vi "ExpStateLoadBridge.vi"(3 "Error In":errorcluster, 5 "Experiment State IN":T1={"error"={"status"=FALSE, "code"=0, "source"=""}, "Digitizer DAQmx Tasks"={"TaskArray"=[]}, "Digitizer Settings"={"Channel Settings"=[], "Card Settings"=[]}, "Synchronization Settings"={"Synchronizer"="PXI1Slot2", "source terminal"="GlobalSoftwareTrigger"}, "Digitizer Data"=[], "Next Shot#"="0", "System Message"="", "User Shot Notes"="", "Timing Settings"={"Timing Card Settings"=[], "Timing Channel Settings"=[[{"Delay (s)"=2.559999942779541, "Pulse width (s)"=0.009999999776482582, "Active"=TRUE, "Channel Name"="Fiber 8", "counter"="PXI1Slot8/ctr7", "FrontPanelTime"=2.559999942779541}]]}, "Timing Tasks"={"TaskArray"=[]}, "Tree"="0", "Time Card/Channels"=[2, 8], "DAQ Card/Channels"=[3, 8], "Program Version"=""} {"Timing Settings"."Timing Channel Settings"."FrontPanelTime" format="%.3p"; "Timing Settings"."Timing Channel Settings"."Pulse width (s)" format="%.3p"; "Timing Settings"."Timing Channel Settings"."Delay (s)" format="%.3p"; "Digitizer Settings"."Card Settings"."Global Edge Type" items=["Rising"=10280, "Falling"=10171]; "Digitizer Settings"."Card Settings"."Sample Rate" format="%#_3p"}) -> (0 "Initialized DAQ Array":T11(array[cluster]) {"Card Settings"."Start Time" format="%#_3p"; "Card Settings"."End Time" format="%#_3p"; "Card Settings"."Rate" format="%#_3p"}, 1 "Initialized Timing Array":T12[](array[typedef]) {"Timing Sequence"."Dt" format="%_3p"; "Timing Sequence"."Time" format="%_3p"}, 2 "Experiment State OUT":T1={"error"={"status"=FALSE, "code"=0, "source"=""}, "Digitizer DAQmx Tasks"={"TaskArray"=[]}, "Digitizer Settings"={"Channel Settings"=[], "Card Settings"=[]}, "Synchronization Settings"={"Synchronizer"="PXI1Slot2", "source terminal"="GlobalSoftwareTrigger"}, "Digitizer Data"=[], "Next Shot#"="0", "System Message"="", "User Shot Notes"="", "Timing Settings"={"Timing Card Settings"=[], "Timing Channel Settings"=[[{"Delay (s)"=2.559999942779541, "Pulse width (s)"=0.009999999776482582, "Active"=TRUE, "Channel Name"="Fiber 8", "counter"="PXI1Slot8/ctr7", "FrontPanelTime"=2.559999942779541}]]}, "Timing Tasks"={"TaskArray"=[]}, "Tree"="0", "Time Card/Channels"=[2, 8], "DAQ Card/Channels"=[3, 8], "Program Version"=""} {"Timing Settings"."Timing Channel Settings"."FrontPanelTime" format="%.3p"; "Timing Settings"."Timing Channel Settings"."Pulse width (s)" format="%.3p"; "Timing Settings"."Timing Channel Settings"."Delay (s)" format="%.3p"; "Digitizer Settings"."Card Settings"."Global Edge Type" items=["Rising"=10280, "Falling"=10171]; "Digitizer Settings"."Card Settings"."Sample Rate" format="%#_3p"})   [LabVIEW 2013]
uses:
  Controls/TimingControl.ctl
  Controls/TimingControlChannel.ctl
  Controls/DAQ Card Channel Array.ctl
  Controls/DAQ Channel Settings.ctl
  Controls/DAQ Card Settings.ctl
  Controls/ExperimentStateCluster.ctl
  Controls/DigitizerSettingsChannelSettings.ctl
  Controls/DigitizerSettingsCardSettingsArray.ctl
  Controls/DigitizerSettingsCardSettings.ctl
  Controls/TimingSettings.ctl
  Controls/TimingCardSettings.ctl
  Controls/TimingChannelSettings.ctl
  Controls/DAQ Card-Channel Settings.ctl
panel:
  # "Sampling Rate [1/s]"
  # "Start Time [s]"
  # "End Time [s]"
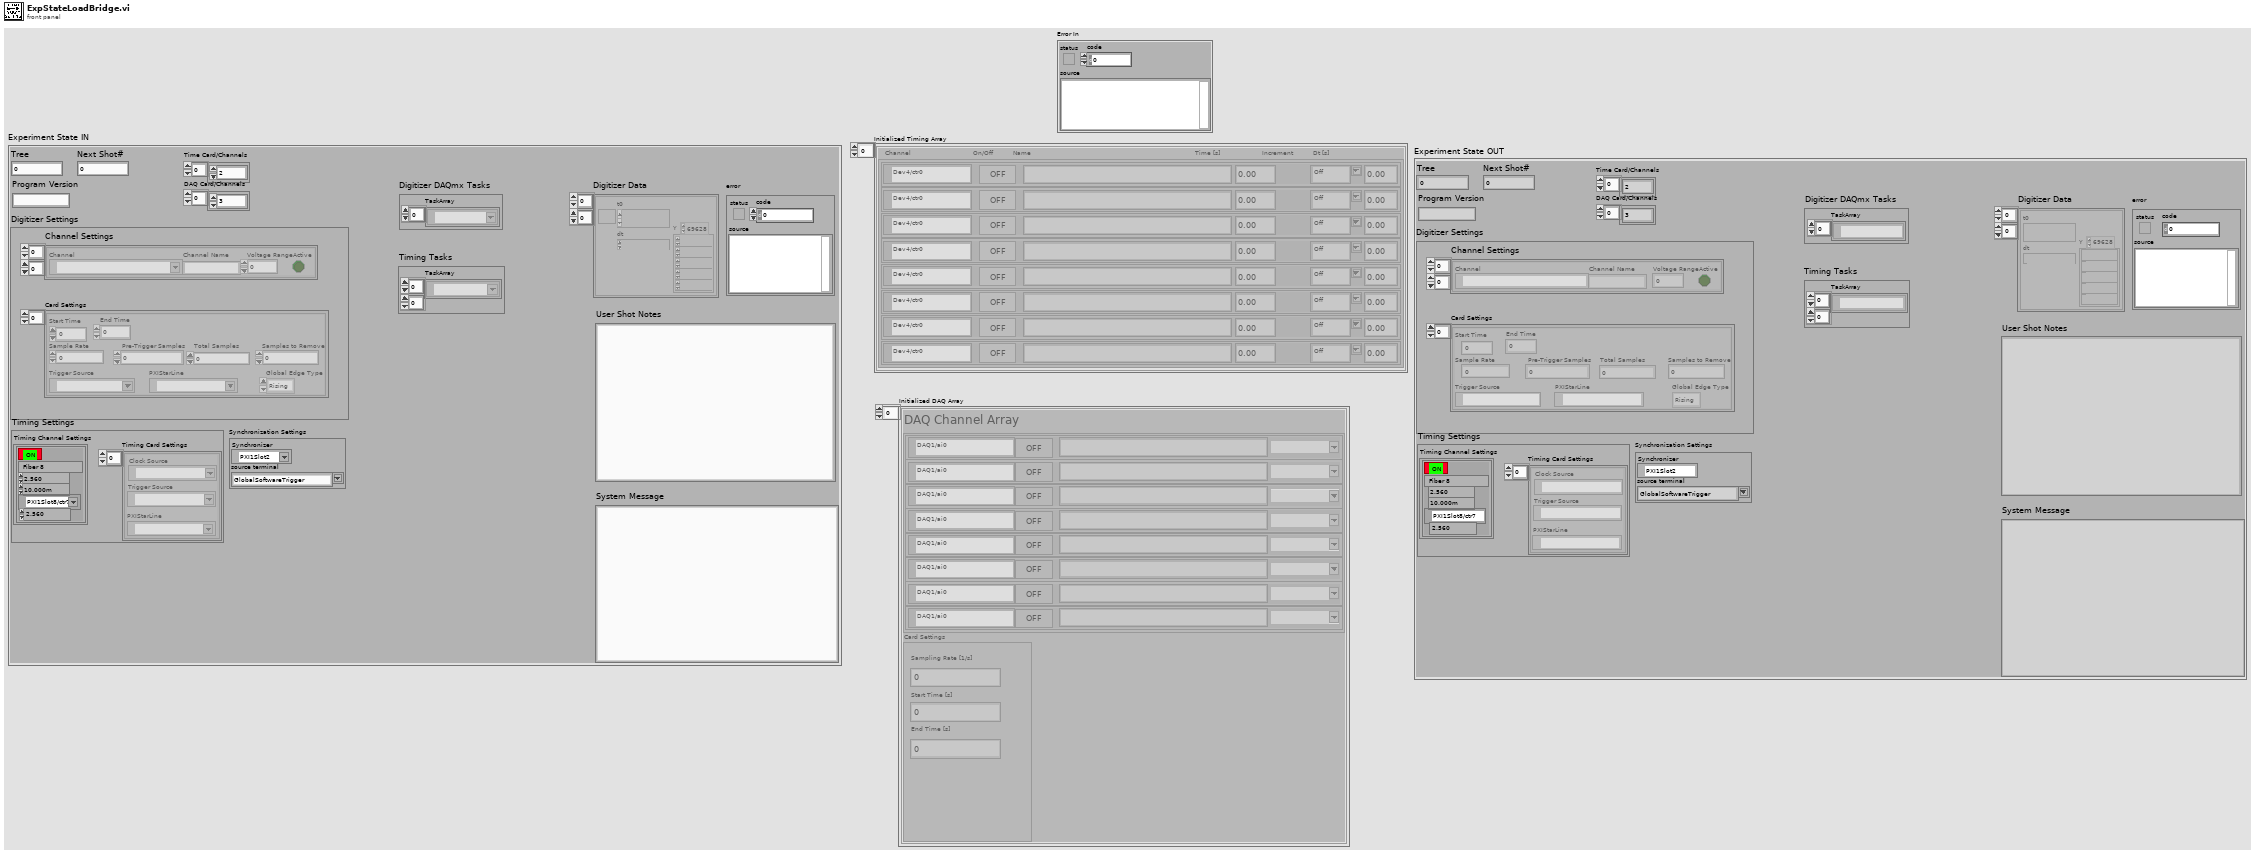
[diagram p1: front panel]
types:
  T1 = typedef "ExperimentStateCluster.ctl" = cluster{"error":errorcluster, "Digitizer DAQmx Tasks":cluster{"TaskArray":refnum<k21>[]}, "Digitizer Settings":cluster{"Channel Settings":T2[][], "Card Settings":T3}, "Synchronization Settings":cluster{"Synchronizer":refnum<k15>, "source terminal":string}, "Digitizer Data":waveform(dbl)[][], "Next Shot#":string, "System Message":string, "User Shot Notes":string, "Timing Settings":T5, "Timing Tasks":cluster{"TaskArray":refnum<k21>[][]}, "Tree":string, "Time Card/Channels":i32[], "DAQ Card/Channels":i32[], "Program Version":string}
  T2 = typedef "DigitizerSettingsChannelSettings.ctl" = cluster{"Channel":tag, "Channel Name":string, "Voltage Range":dbl, "Active":bool}
  T3 = typedef "DigitizerSettingsCardSettingsArray.ctl" = T4[]
  T4 = typedef "DigitizerSettingsCardSettings.ctl" = cluster{"Start Time":dbl, "End Time":dbl, "Sample Rate":dbl, " Pre-Trigger Samples":u32, "Total Samples":i32, "Samples to Remove":u32, "Trigger Source":tag, "Global Edge Type":i32, "PXIStarLine":tag}
  T5 = typedef "TimingSettings.ctl" = cluster{"Timing Card Settings":T6[], "Timing Channel Settings":T7[][]}
  T6 = typedef "TimingCardSettings.ctl" = cluster{"Trigger Source":tag, "Clock Source":tag, "PXIStarLine":tag}
  T7 = typedef "TimingChannelSettings.ctl" = cluster{"Delay (s)":dbl, "Pulse width (s)":dbl, "Active":bool, "Channel Name":string, "counter":tag, "FrontPanelTime":dbl}
  T8 = typedef "DAQ Card Channel Array.ctl" = T9[]
  T9 = typedef "DAQ Channel Settings.ctl" = cluster{"Active":bool, "Channel Name":string, "Channel":tag, "Voltage Range":string}
  T10 = typedef "DAQ Card Settings.ctl" = cluster{"Rate":dbl, "End Time":dbl, "Start Time":dbl}
  T11 = cluster{"DAQ Channel Array":T8, "Card Settings":T10}[]
  T12 = typedef "TimingControl.ctl" = cluster{"Timing Sequence":T13[]}
  T13 = typedef "TimingControlChannel.ctl" = cluster{"Active":bool, "counter":tag, "Channel Name":string, "Time":dbl, "Increment":string, "Dt":dbl}
  T14 = typedef "DAQ Card-Channel Settings.ctl" = cluster{"DAQ Channel Array":T8, "Card Settings":T10}
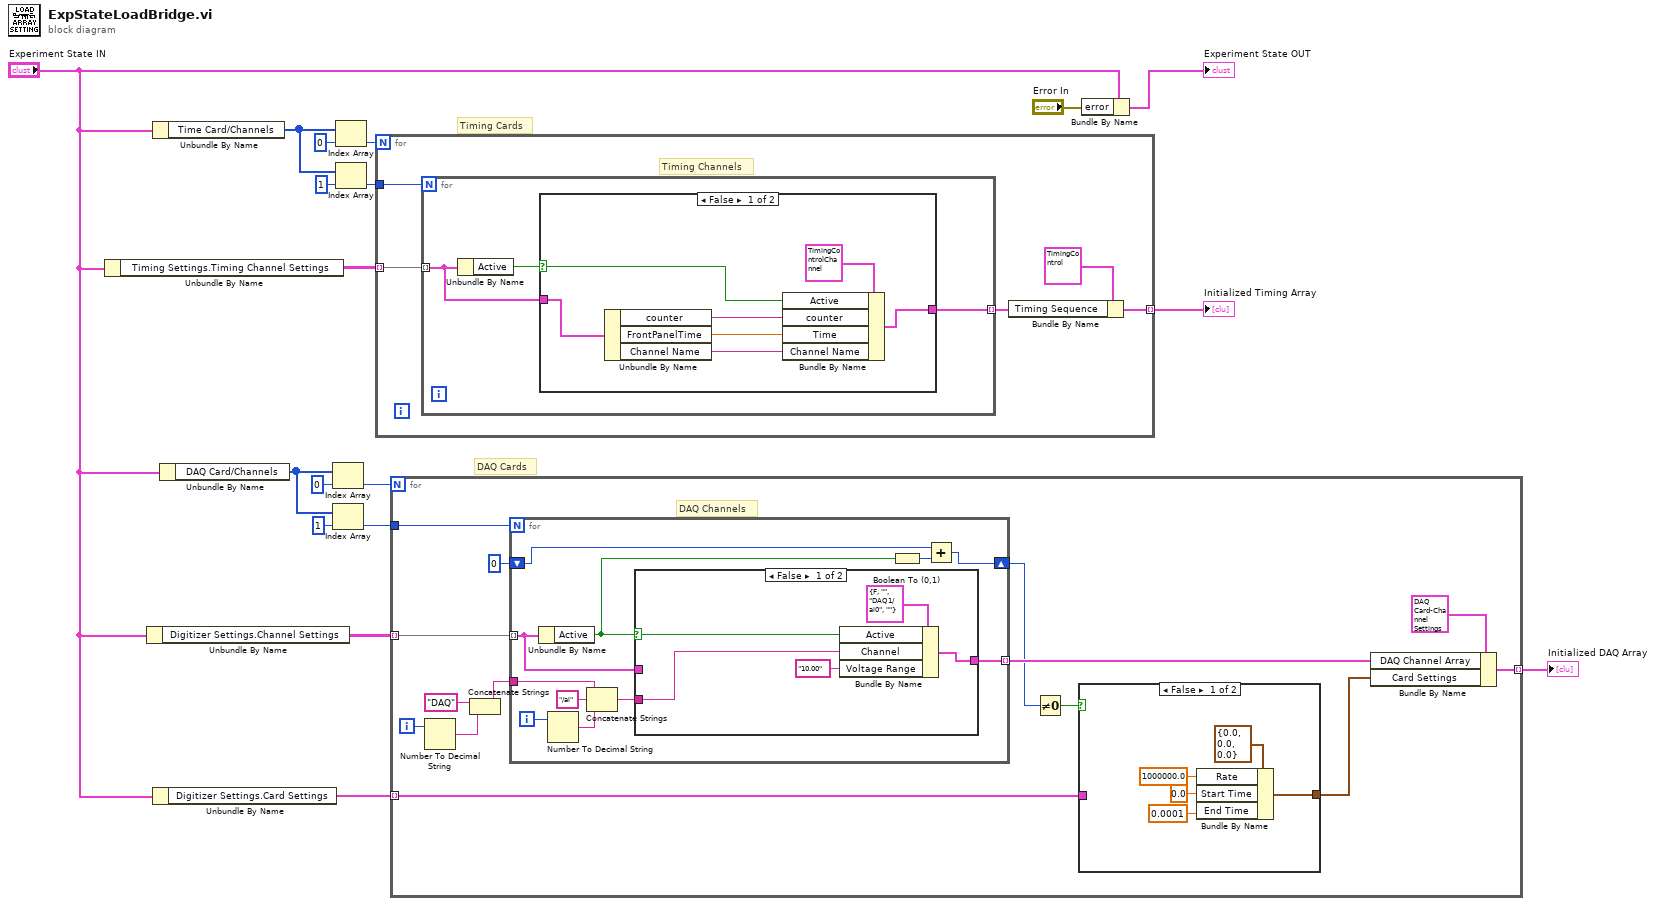
[diagram p0: block diagram]
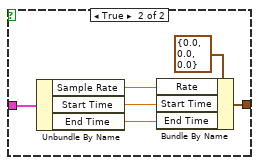
[diagram p2: hidden frame]
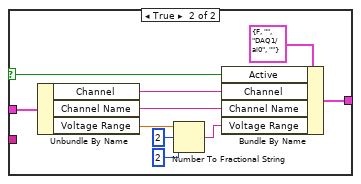
[diagram p3: hidden frame]
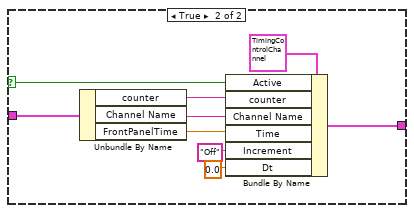
[diagram p4: hidden frame]
diagram:
  # "DAQ Cards"
  # "Timing Cards"
  n1 = Unbundle By Name("Experiment State IN") -> ("Timing Settings.Timing Channel Settings"=w11:T7[][])
  n2 = Unbundle By Name("Experiment State IN") -> ("Digitizer Settings.Channel Settings"=w5:T2[][])
  n3 = Unbundle By Name("Experiment State IN") -> ("Time Card/Channels"=w13:i32[])
  n4 = Unbundle By Name("Experiment State IN") -> ("Digitizer Settings.Card Settings"=w4:T3)
  n5 = Unbundle By Name("Experiment State IN") -> ("DAQ Card/Channels"=w8:i32[])
  n6 = Index Array(array=w8, index=0) -> (element=w7:i32)
  n7 = Index Array(array=w8, index=1) -> (element=w6:i32)
  n8 = Index Array(array=w13, index=0) -> (element=w16:i32)
  n9 = Index Array(array=w13, index=1) -> (element=w12:i32)
  n10 = for {
    N: w16 -> [_]
    tunnel: [w23] -> w18 mode=indexing
    tunnel: w12 -> [w20]
    tunnel: w11 -> [w19] mode=indexing
    # "Timing Channels"
    n11 = for {
      N: w20 -> [_]
      tunnel: [w25] -> w21 mode=indexing
      tunnel: w19 -> [w24] mode=indexing
      n12 = Unbundle By Name(w24) -> ("Active"=w26:bool)
      n13 = case shown="False" w26 {
        selector: w26 -> [w32 w38]
        tunnel: [w31 w39] -> w25
        tunnel: w24 -> [w30 w37]
        frame False {
          n14 = Unbundle By Name(w30) -> ("counter"=w29:tag, "FrontPanelTime"=w28:dbl, "Channel Name"=w27:string)
          n15 = Bundle By Name(cluster=T13 {"Active"=FALSE, "counter"="PXI1Slot9/ctr7", "Channel Name"="", "Time"=0.0, "Increment"="Off", "Dt"=0.0} ("Counters"), "Active"=w32, "counter"=w29, "Time"=w28, "Channel Name"=w27) -> (w31:T13)
        }
        frame True {
          n16 = Unbundle By Name(w37) -> ("counter"=w36:tag, "Channel Name"=w35:string, "FrontPanelTime"=w34:dbl)
          n17 = Bundle By Name(cluster=T13 {"Active"=FALSE, "counter"="PXI1Slot9/ctr7", "Channel Name"="", "Time"=0.0, "Increment"="Off", "Dt"=0.0} ("Counters"), "Active"=w38, "counter"=w36, "Channel Name"=w35, "Time"=w34, "Increment"="Off", "Dt"=0.0) -> (w39:T13)
        }
      }
    }
    n18 = Bundle By Name(cluster=T12 {"Timing Sequence"=[{"Active"=FALSE, "counter"="PXI1Slot9/ctr7", "Channel Name"="", "Time"=0.0, "Increment"="Off", "Dt"=0.0}, {"Active"=FALSE, "counter"="Dev4/ctr0", "Channel Name"="", "Time"=0.0, "Increment"="Off", "Dt"=0.0}, {"Active"=FALSE, "counter"="Dev4/ctr0", "Channel Name"="", "Time"=0.0, "Increment"="Off", "Dt"=0.0}, {"Active"=FALSE, "counter"="Dev4/ctr0", "Channel Name"="", "Time"=0.0, "Increment"="Off", "Dt"=0.0}, {"Active"=FALSE, "counter"="Dev4/ctr0", "Channel Name"="", "Time"=0.0, "Increment"="Off", "Dt"=0.0}, {"Active"=FALSE, "counter"="Dev4/ctr0", "Channel Name"="", "Time"=0.0, "Increment"="Off", "Dt"=0.0}, {"Active"=FALSE, "counter"="Dev4/ctr0", "Channel Name"="", "Time"=0.0, "Increment"="Off", "Dt"=0.0}, {"Active"=FALSE, "counter"="Dev4/ctr0", "Channel Name"="", "Time"=0.0, "Increment"="Off", "Dt"=0.0}]} ("Cluster"), "Timing Sequence"=w21) -> (w23:T12)
  }
  "Initialized Timing Array" <- w18
  n19 = for {
    N: w7 -> [_]
    tunnel: [w56] -> w17 mode=indexing
    tunnel: w6 -> [w53]
    tunnel: w5 -> [w52] mode=indexing
    tunnel: w4 -> [w47] mode=indexing
    i -> [w44]
    # "DAQ Channels"
    n20 = Number To Decimal String(number=w44) -> (decimal integer string=w46:string)  [unwired: 1 in]
    n21 = Concatenate Strings("DAQ", w46) -> (w43:string)
    n22 = for {
      N: w53 -> [_]
      tunnel: [w78] -> w54 mode=indexing
      tunnel: w52 -> [w77] mode=indexing
      shift-right: [w73] -> w49
      shift-left: 0 -> [w74]
      tunnel: w43 -> [w70]
      i -> [w69]
      n23 = Unbundle By Name(w77) -> ("Active"=w75:bool)
      n24 = Number To Decimal String(number=w69) -> (decimal integer string=w72:string)  [unwired: 1 in]
      n25 = Concatenate Strings(w70, "/ai" ("string"), w72) -> (w68:string)
      n26 = case shown="False" w75 {
        selector: w75 -> [w81 w91]
        tunnel: [w82 w93] -> w78
        tunnel: w77 -> [_ w90]
        tunnel: w68 -> [w79 _]
        frame False {
          n27 = Bundle By Name(cluster=T9 {"Active"=FALSE, "Channel Name"="", "Channel"="DAQ1/ai0", "Voltage Range"=""} ("Counters"), "Active"=w81, "Channel"=w79, "Voltage Range"="10.00") -> (w82:T9)
        }
        frame True {
          n28 = Unbundle By Name(w90) -> ("Channel"=w88:tag, "Channel Name"=w89:string, "Voltage Range"=w86:dbl)
          n29 = Number To Fractional String(number=w86, width (-)=i16 2, precision (6)=i16 2) -> (F-format string=w87:string)  [unwired: 1 in]
          n30 = Bundle By Name(cluster=T9 {"Active"=FALSE, "Channel Name"="", "Channel"="DAQ1/ai0", "Voltage Range"=""} ("Counters"), "Active"=w91, "Channel"=w88, "Channel Name"=w89, "Voltage Range"=w87) -> (w93:T9)
        }
      }
      n31 = Boolean To (0,1)(Boolean=w75) -> (0, 1=w76:i16)
      n32 = Add(x=w74, y=w76) -> (x+y=w73:i32)
    }
    n33 = Not Equal To 0?(x=w49) -> (x != 0?=w50:bool)
    n34 = case shown="False" w50 {
      tunnel: [w58 w66] -> w48
      tunnel: w47 -> [_ w65]
      frame False {
        n35 = Bundle By Name(cluster=T10 {"Rate"=0.0, "End Time"=0.0, "Start Time"=0.0} ("Card Settings"), "Rate"=1000000.0, "Start Time"=0.0, "End Time"=0.0001) -> (w58:T10)
      }
      frame True {
        n36 = Unbundle By Name(w65) -> ("Sample Rate"=w62:dbl, "Start Time"=w63:dbl, "End Time"=w64:dbl)
        n37 = Bundle By Name(cluster=T10 {"Rate"=0.0, "End Time"=0.0, "Start Time"=0.0} ("Card Settings"), "Rate"=w62, "Start Time"=w63, "End Time"=w64) -> (w66:T10)
      }
    }
    n38 = Bundle By Name(cluster=T14 {"DAQ Channel Array"=[{"Active"=FALSE, "Channel Name"="", "Channel"="DAQ1/ai0", "Voltage Range"=""}, {"Active"=FALSE, "Channel Name"="", "Channel"="DAQ1/ai0", "Voltage Range"=""}, {"Active"=FALSE, "Channel Name"="", "Channel"="DAQ1/ai0", "Voltage Range"=""}, {"Active"=FALSE, "Channel Name"="", "Channel"="DAQ1/ai0", "Voltage Range"=""}, {"Active"=FALSE, "Channel Name"="", "Channel"="DAQ1/ai0", "Voltage Range"=""}, {"Active"=FALSE, "Channel Name"="", "Channel"="DAQ1/ai0", "Voltage Range"=""}, {"Active"=FALSE, "Channel Name"="", "Channel"="DAQ1/ai0", "Voltage Range"=""}, {"Active"=FALSE, "Channel Name"="", "Channel"="DAQ1/ai0", "Voltage Range"=""}], "Card Settings"={"Rate"=100.0, "End Time"=0.0, "Start Time"=0.0}} ("Cluster"), "DAQ Channel Array"=w54, "Card Settings"=w48) -> (w56:T14)
  }
  "Initialized DAQ Array" <- w17
  n39 = Bundle By Name(cluster="Experiment State IN", "error"="Error In") -> (→"Experiment State OUT":T1)
